vi "2.4.vi"() -> ()   [LabVIEW 2017]
panel:
  out "y":dbl
  in  "x":dbl
  in  "b":dbl
  in  "k":dbl
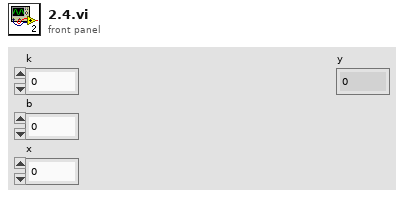
[diagram p1: front panel]
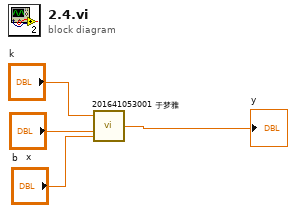
[diagram p0: block diagram]
diagram:
  n1 = call "201641053001 于梦雅.vi"("b"="b", "x"="x", "k"="k") -> ("y"=→"y":dbl)
